vi "carga.vi"() -> ()   [LabVIEW 2016]
panel:
  in  "Reset (F)":bool
  in  "VISA":refnum<visa-resource-name>="GPIB::05::INSTR"
  in  "OUTPUT":bool caption="Boolean"
  in  "stop":bool
  out "Output Current":dbl format="%.4f"
  out "Output Voltage":dbl format="%.4f"
  in  "Current Limit":dbl format="%.4f"
  in  "Voltage Limit":dbl format="%.4f"
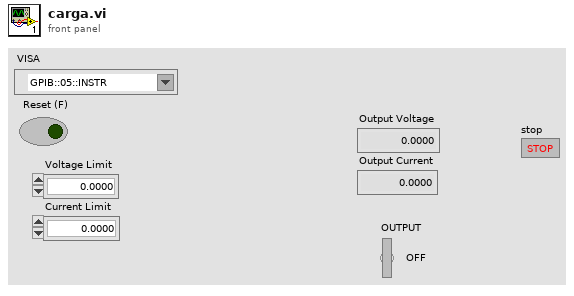
[diagram p1: front panel]
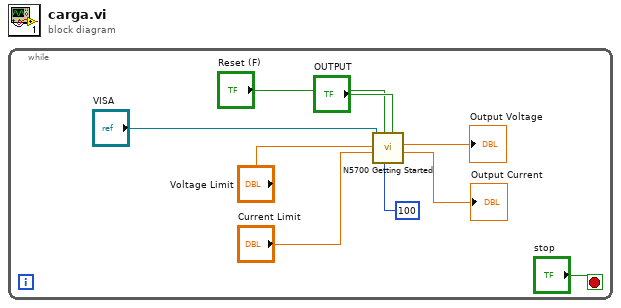
[diagram p0: block diagram]
diagram:
  n1 = while {
    stop <- "stop" stop-if-true
    n2 = call <instrlib>:"N5700 Getting Started.vi"("Output On (T)"="OUTPUT", "Settle (0 mS)"=u32 100, "Reset (F)"="Reset (F)", "Current Limit"="Current Limit", "Voltage Limit"="Voltage Limit", "VISA"="VISA") -> ("Output Current"=→"Output Current":dbl, "Output Voltage"=→"Output Voltage":dbl)  [unwired: 2 in, 2 out]
  }
